vi "I16 Array To FXP-SGL Array.vi"(2 "小数位数":i32=2, 3 "I16 Array":u16[](array[numeric])=[52429, 17142, 3072, 17799, 35226, 17559] format="%04x") -> (0 "SGL Array":sgl[](array[numeric]) format="%.3f", 1 "元素0":sgl)   [LabVIEW 2018]
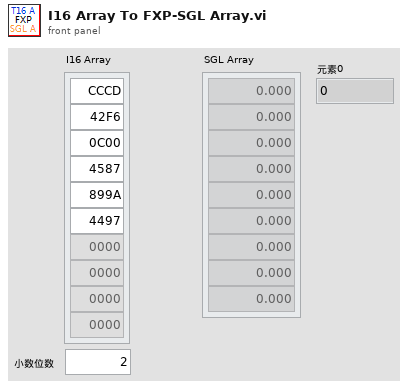
[diagram p1: front panel]
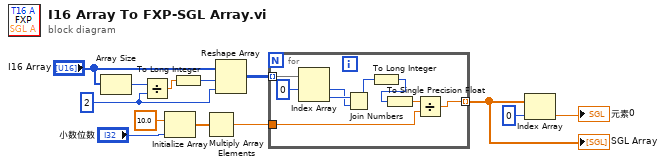
[diagram p0: block diagram]
diagram:
  w8 = 2 ("维数大小")
  n1 = Array Size(array="I16 Array") -> (size(s)=w11:i32)
  n2 = Divide(x=w11, y=w8) -> (x/y=w10:dbl)
  n3 = Initialize Array(sgl 10.0 ("元素"), "小数位数") -> (w2:sgl[])
  n4 = To Long Integer(number=w10) -> (32bit integer=w9:i32)
  n5 = Multiply Array Elements(1:w2) -> (0:w1:sgl)
  n6 = Reshape Array("I16 Array", w9, w8) -> (w13:u16[][])
  n7 = for {
    tunnel: w13 -> [w22] mode=indexing
    tunnel: [w17] -> w6 mode=indexing
    tunnel: w1 -> [w18]
    n8 = Index Array(array=w22, index #1=0 ("索引")) -> (element #1=w19:u16, element #2=w20:u16)  [unwired: 1 in]
    n9 = Join Numbers(hi=w20, lo=w19) -> ((hi.lo)=w14:u32)
    n10 = To Long Integer(number=w14) -> (32bit integer=w15:i32)
    n11 = To Single Precision Float(number=w15) -> (single precision float=w16:sgl)
    n12 = Divide(x=w16, y=w18) -> (x/y=w17:sgl)
  }
  "SGL Array" <- w6
  n13 = Index Array(array=w6, index=0 ("索引")) -> (element=→"元素0":sgl)
